vi "Modules Selector individual.vi"(8 "Module In Dependencies? in":bool[](array[boolean]), 10 "Modules Types In":T2[](array[typedef]), 11 "DQMH Modules In":refnum<vi>[](array[refnum])) -> (0 "Module In Dependencies? Out":bool=TRUE, 2 "Modules Type Out":T2, 3 "DQMH Module Out":refnum<vi>, 4 "Scan?":bool)   [LabVIEW 2019, in "Panther Dashboard.lvlib"]
uses:
  Panther Dashboard.lvlib
  Module type--enum.ctl
  Module to scan--cluster.ctl
panel:
  in  "DQMH Modules found in Project":T1[](array[typedef])
  in  "Scan Selection":bool caption="Scan Selected Module"
  # "Only one Module can be selected, make sure it is not already listed\nif already listed you'll have to delete the duplicate"
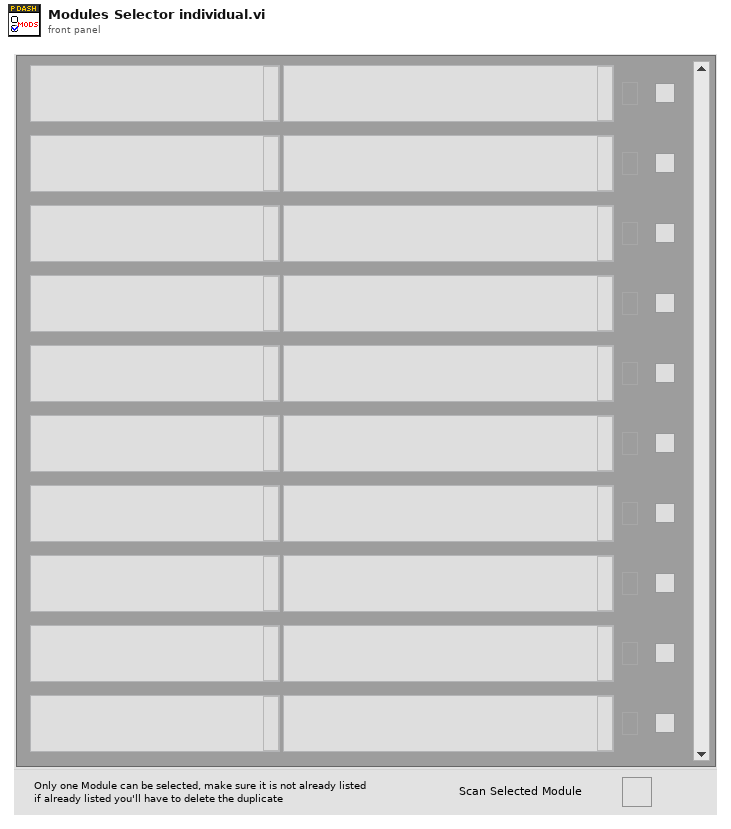
[diagram p1: front panel]
types:
  T1 = typedef "Panther Dashboard.lvlib/Module to scan--cluster.ctl" = cluster{"Module Name":string, "Description":string, "Scan?":bool, "Dependency":bool}
  T2 = typedef "Panther Dashboard.lvlib/Module type--enum.ctl" = enum16{"Singleton", "Cloneable"}
  T3 = enum32{"Invalid", "Standard", "Closed", "Hidden", "Minimized", "Maximized"}
  T4 = enum8{"Enabled", "Disabled", "Disabled and Grayed Out"}
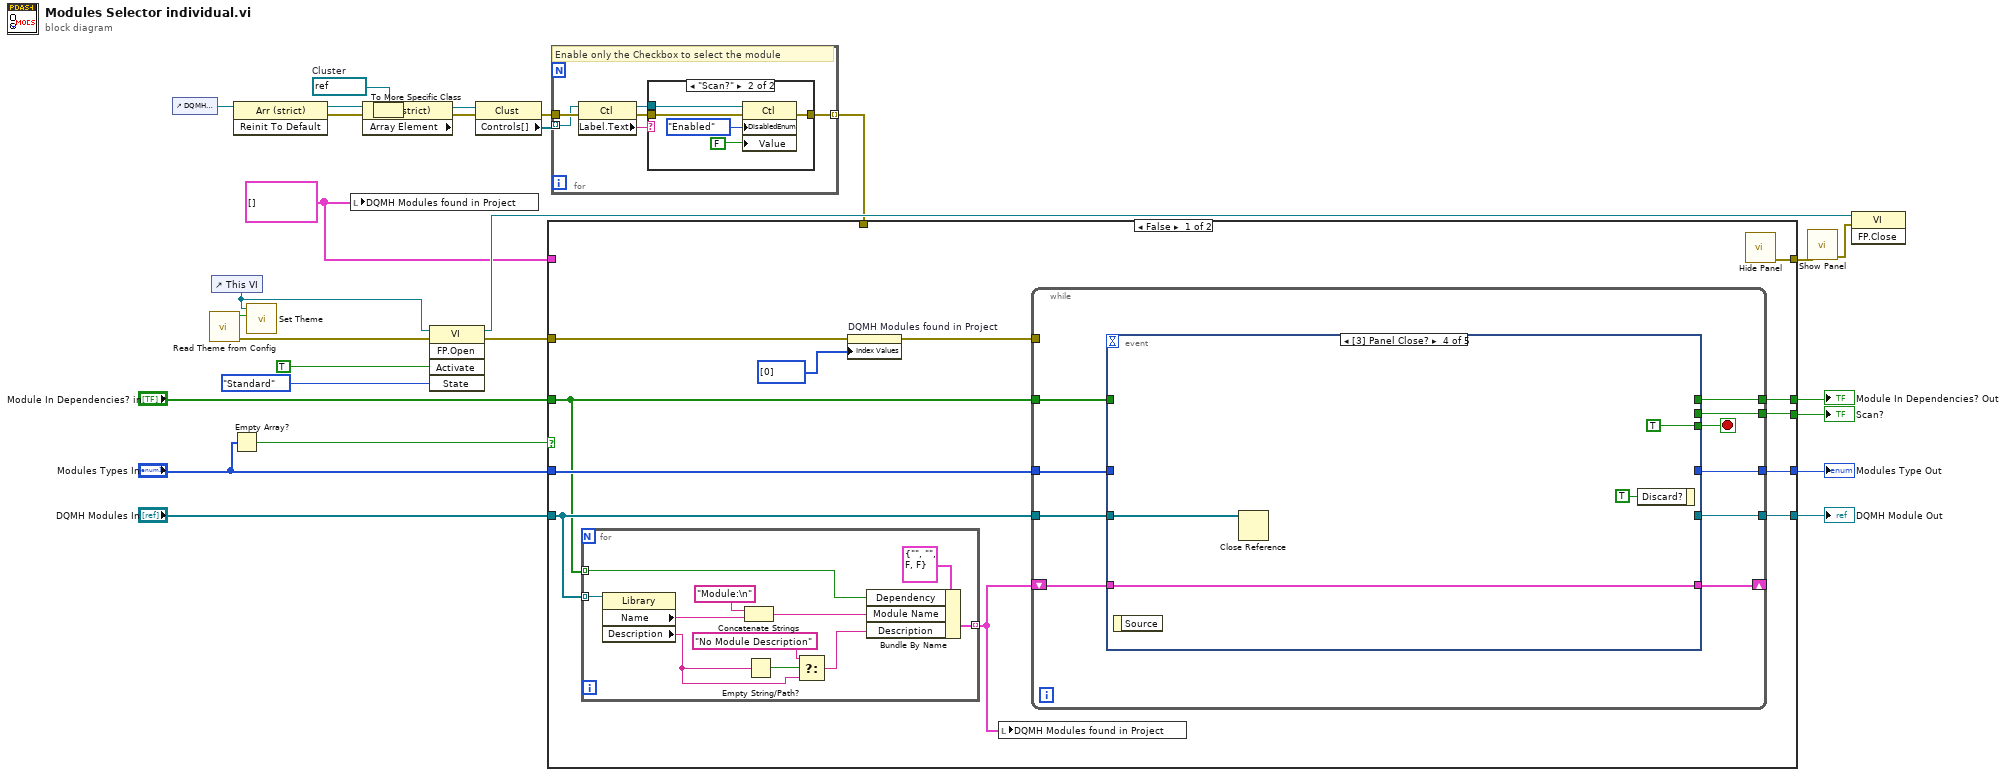
[diagram p0: block diagram]
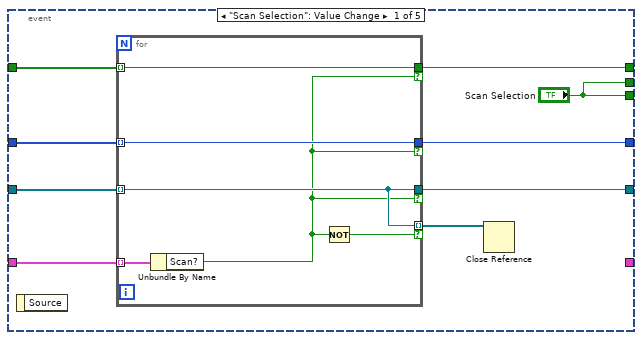
[diagram p2: hidden frame]
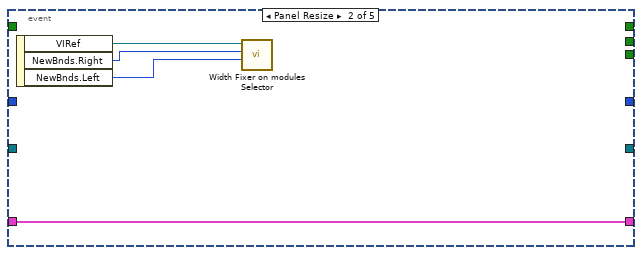
[diagram p3: hidden frame]
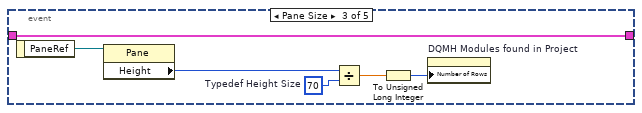
[diagram p4: hidden frame]
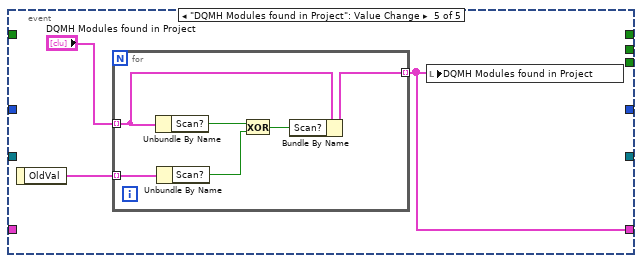
[diagram p5: hidden frame]
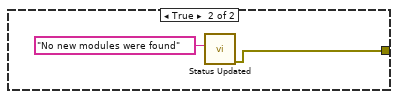
[diagram p6: hidden frame]
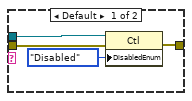
[diagram p7: hidden frame]
diagram:
  w5 = refnum<vi> refnum  # Cluster
  w10 = T1[] [] ("DQMH Modules found in Project")
  n1 = control-ref of="DQMH Modules found in Project"() -> (w9:refnum<vi>)
  n2 = call "Read Theme from Config.vi"() -> ("error out"=w29:errorcluster, "Theme"=w16:bool)  [unwired: 10 in]
  n3 = control-ref of="This VI"() -> (w14:refnum<vi>)
  n4 = Empty Array?(array="Modules Types In") -> (empty?=w15:bool)
  n5 = invoke class="Arr (strict)" method="Reinit To Default"(reference=w9) -> (reference out=w3:refnum<vi>, error out=w24:errorcluster)  [unwired: 2 in, 1 out]
  n6 = call "Set Theme.vi"("Dark?"=w16, "VI in"=w14) -> ()  [unwired: 10 in]
  n7 = local write "DQMH Modules found in Project"(w10) -> ()
  n8 = property class="Arr (strict)"(reference=w3, error in=w24) -> (error out=w27:errorcluster, "Array Element"=w8:refnum<vi>)  [unwired: 1 out]
  n9 = To More Specific Class(target class=w5, reference=w8, error in=w27) -> (specific class reference=w7:refnum<vi>, error out=w26:errorcluster)
  n10 = invoke class="VI" method="FP.Open"(reference=w14, error in=w29, "Activate"=TRUE ("Activate?"), "State"=T3."Standard") -> (reference out=w11:refnum<vi>, error out=w28:errorcluster)  [unwired: 1 in, 3 out]
  n11 = property class="Clust"(reference=w7, error in=w26) -> (error out=w25:errorcluster, "Controls[]"=w6:refnum<vi>[])  [unwired: 1 out]
  n12 = for {
    tunnel: w6 -> [w32] mode=indexing
    tunnel: w25 -> [w35]
    tunnel: [w33] -> w4 mode=indexing
    # "Enable only the Checkbox to select the module"
    n13 = property class="Ctl"(reference=w32, error in=w35) -> (reference out=w30:refnum<vi>, error out=w34:errorcluster, "Label.Text"=w31:string)
    n14 = case shown="\"Scan?\"" w31 {
      tunnel: w30 -> [w37 w42]
      tunnel: w34 -> [w39 w44]
      tunnel: [w38 w43] -> w33
      frame Default {
        n15 = property class="Ctl"(reference=w37, error in=w39, "DisabledEnum"=T4."Disabled" ("Disabled")) -> (error out=w38:errorcluster)  [unwired: 1 out]
      }
      frame "Scan?" {
        n16 = property class="Ctl"(reference=w42, error in=w44, "DisabledEnum"=T4."Enabled" ("Disabled"), "Value"=FALSE) -> (error out=w43:errorcluster)  [unwired: 1 out]
      }
    }
  }
  n17 = case shown="False" w15 {
    tunnel: "DQMH Modules In" -> [w50 _]
    tunnel: [w53 _] -> w20
    tunnel: "Modules Types In" -> [w52 _]
    tunnel: [w51 _] -> w22
    tunnel: w28 -> [w55 _]
    tunnel: [w56 w117] -> w2
    tunnel: "Module In Dependencies? in" -> [w46 _]
    tunnel: [w47 _] -> w18
    tunnel: [w45 _] -> w17
    tunnel: w10 -> [_ _]
    tunnel: w4 -> [_ _]
    frame False {
      n18 = for {
        tunnel: w50 -> [w115] mode=indexing
        tunnel: [w114] -> w49 mode=indexing
        tunnel: w46 -> [w105] mode=indexing
        n19 = property class="Library"(reference=w115) -> ("Name"=w112:string, "Description"=w110:string)  [unwired: 1 in, 2 out]
        n20 = Concatenate Strings("Module:\n" ("string"), w112) -> (w107:string)
        n21 = Empty String/Path?(string/path=w110) -> (empty?=w111:bool)
        n22 = Select(t="No Module Description", s=w111, f=w110) -> (s? t:f=w109:string)
        n23 = Bundle By Name(cluster=T1 {"Module Name"="", "Description"="", "Scan?"=FALSE, "Dependency"=FALSE} ("Module"), "Dependency"=w105, "Module Name"=w107, "Description"=w109) -> (w114:T1)
      }
      n24 = property on="DQMH Modules found in Project" class="Arr (strict)"(error in=w55, "Index Values"=u32[] [0]) -> (error out=w54:errorcluster)  [unwired: 1 in, 1 out]
      n25 = local write "DQMH Modules found in Project"(w49) -> ()
      n26 = while {
        shift-right: [w65] -> _
        shift-left: w49 -> [w66]
        tunnel: w50 -> [w64]
        tunnel: [w63] -> w53
        tunnel: w52 -> [w62]
        tunnel: [w61] -> w51
        tunnel: w54 -> [_]
        tunnel: w46 -> [w60]
        tunnel: [w59] -> w47
        tunnel: [w57] -> w45
        stop <- w58 stop-if-true
        n27 = event shown="[3] Panel Close?" {
          selector: _ -> [_ _ _ _ _]
          dyn-events: _ -> [_ _ _ _ _]
          timeout: _ -> [_ _ _ _ _]
          tunnel: w66 -> [w75 w85 w87 w93 _]
          tunnel: ["Scan Selection" _ _ TRUE ("All") _] -> w58
          tunnel: [_ w85 w87 w93 w97] -> w65
          tunnel: [w71 _ _ _ _] -> w63
          tunnel: w64 -> [w73 _ _ w94 _]
          tunnel: w62 -> [w74 _ _ _ _]
          tunnel: [w72 _ _ _ _] -> w61
          tunnel: w60 -> [w69 _ _ _ _]
          tunnel: [w68 _ _ _ _] -> w59
          tunnel: ["Scan Selection" _ _ _ _] -> w57
          event "Scan Selection": Value Change {
            n28 = event-data() -> ()  [unwired: 1 in, 1 out]
            n29 = for {
              tunnel: w75 -> [w81] mode=indexing
              tunnel: w74 -> [w80] mode=indexing
              tunnel: w73 -> [w79] mode=indexing
              tunnel: [w80] -> w72 if=w76
              tunnel: [w79] -> w71 if=w76
              tunnel: [w79] -> w70 mode=indexing if=w78
              tunnel: w69 -> [w77] mode=indexing
              tunnel: [w77] -> w68 if=w76
              n30 = Unbundle By Name(w81) -> ("Scan?"=w76:bool)
              n31 = Not(x=w76) -> (.not. x?=w78:bool)
            }
            n32 = Close Reference(reference=w70) -> ()  [unwired: 1 in, 1 out]
          }
          event Panel Resize {
            n33 = event-data() -> ("VIRef"=w84:refnum<vi>, "NewBnds.Right"=w82:i16, "NewBnds.Left"=w83:i16)  [unwired: 1 in]
            n34 = call "Width Fixer on modules Selector.vi"("Left"=w83, "Right"=w82, "VI in"=w84) -> ()  [unwired: 9 in]
          }
          event Pane Size {
            w89 = u32 70  # Typedef Height Size
            n35 = event-data() -> ("PaneRef"=w91:refnum<vi>)  [unwired: 1 in]
            n36 = property class="Pane"(reference=w91) -> ("Height"=w90:u32)  [unwired: 1 in, 2 out]
            n37 = Divide(x=w90, y=w89) -> (x/y=w88:dbl)
            n38 = To Unsigned Long Integer(number=w88) -> (unsigned 32bit integer=w86:u32)
            n39 = property on="DQMH Modules found in Project" class="Arr (strict)"("Number of Rows"=w86) -> ()  [unwired: 2 in, 2 out]
          }
          event Panel Close? {
            n40 = event-data() -> ()  [unwired: 1 in, 1 out]
            n41 = Close Reference(reference=w94) -> ()  [unwired: 1 in, 1 out]
            n42 = event-data("Discard?"=TRUE) -> ()  [unwired: 1 in, 1 out]
          }
          event "DQMH Modules found in Project": Value Change {
            n43 = event-data() -> ("OldVal"=w96:T1[])  [unwired: 1 in]
            n44 = for {
              tunnel: "DQMH Modules found in Project" -> [w103] mode=indexing
              tunnel: [w102] -> w97 mode=indexing
              tunnel: w96 -> [w101] mode=indexing
              n45 = Unbundle By Name(w103) -> ("Scan?"=w104:bool)
              n46 = Unbundle By Name(w101) -> ("Scan?"=w99:bool)
              n47 = Exclusive Or(1:w99, 2:w104) -> (0:w100:bool)
              n48 = Bundle By Name(cluster=w103, "Scan?"=w100) -> (w102:T1)
            }
            n49 = local write "DQMH Modules found in Project"(w97) -> ()
          }
        }
      }
      n50 = call "Hide Panel.vi"() -> ("error out"=w56:errorcluster)  [unwired: 11 in]
    }
    frame True {
      n51 = call "Status Updated.vi"("Status"="No new modules were found") -> ("error out"=w117:errorcluster)  [unwired: 10 in]
    }
  }
  "Modules Type Out" <- w22
  "DQMH Module Out" <- w20
  "Module In Dependencies? Out" <- w18
  "Scan?" <- w17
  n52 = call "Show Panel.vi"("error in (no error)"=w2) -> ("error out"=w1:errorcluster)  [unwired: 10 in]
  n53 = invoke class="VI" method="FP.Close"(reference=w11, error in=w1) -> ()  [unwired: 1 in, 3 out]
